vi "Read Listbox Data.vi"(8 "error in":errorcluster, 11 "Listbox Ref in":refnum<vi>) -> (0 "error out":errorcluster, 1 "Interpret As Unicode":bool, 2 "Value":string[](array[string]), 3 "Listbox Ref out":refnum<vi>)   [LabVIEW 2020, in "G-Unicode.lvlib"]
uses:
  G-Unicode.lvlib
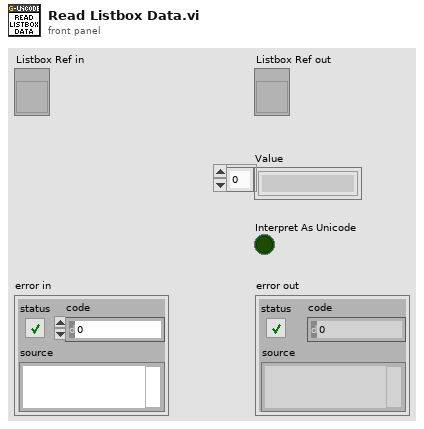
[diagram p1: front panel]
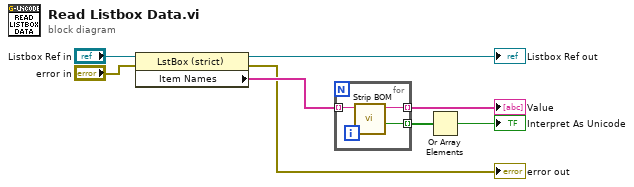
[diagram p0: block diagram]
diagram:
  n1 = property class="LstBox (strict)"(reference="Listbox Ref in", error in="error in") -> (reference out=→"Listbox Ref out":refnum<vi>, error out=→"error out":errorcluster, "Item Names"=w7:string[])
  n2 = for {
    tunnel: w7 -> [w10] mode=indexing
    tunnel: [w11] -> w5 mode=indexing
    tunnel: [w9] -> w8 mode=indexing
    n3 = call "Strip BOM.vi"("String"=w10) -> ("BOM Found"=w9:bool, "String without BOM"=w11:string)  [unwired: 8 in, 1 out]
  }
  "Value" <- w5
  n4 = Or Array Elements(Boolean array=w8) -> (logical OR=→"Interpret As Unicode":bool)
